vi "MT Demodulate CPM.vi"(0 "input complex waveform":T1={"t0"=0.0, "dt"=1.0, "Y"=[]} {"Y" format="%.3f"; "dt" format="%^.2e"; "t0" format="%.4f"}, 5 "CPM system parameters":T3={"samples per symbol (16)"=1, "symbol map"=[]}, 7 "matched filter coefficients":dbl[](array[numeric]) format="%.2f", 9 "synchronization parameters":T4 {"sync sequence" format="%.2f"}, 11 "error in (no error)":errorcluster, 12 "pulse shaping filter coefficients":dbl[](array[numeric]) format="%.2f", 13 "reset? (T)":bool=TRUE) -> (3 "detected complex waveform":T1 {"Y" format="%.3f"; "dt" format="%^.2e"; "t0" format="%.4f"}, 4 "recovered complex waveform":T1 {"Y" format="%.3f"; "dt" format="%^.2e"; "t0" format="%.4f"}, 6 "output bit stream":i8[](array[numeric]), 8 "measurements":T2 {"frequency drift (Hz)" format="%.2f"; "frequency offset (Hz)" format="%.2f"}, 10 "sync found index (symbols)":dbl format="%.4f", 15 "error out":errorcluster)   [LabVIEW 2020, in "niDMT.lvlib"]
doc: "Demodulates a continuous-phase modulation (CPM)-modulated complex baseband waveform and returns the time-aligned demodulated waveform, the demodulated information bit stream, and measurement results obtained during demodulation. This VI attempts to remove carrier and phase offset by locking to the carrier signal."
uses:
  <vilib>/addons/Modulation/niDMT.lvlib
  <vilib>/addons/Modulation/Analog/controls/Complex Data Waveform.ctl
  <vilib>/addons/Modulation/Digital/Support/Controls/CPM System Parameters.ctl
  <vilib>/addons/Modulation/Analog/MT Resample (Complex Cluster).vi
  <vilib>/addons/Modulation/Analog/support/Validators/mod_Fractional Resample Validate.vi
  <vilib>/addons/Modulation/Analog/support/Validators/mod_Check Flush State.vi
  <vilib>/addons/Modulation/Analog/support/mod_FractionalResampler.vi
  <vilib>/addons/Modulation/Analog/support/mod_Integer Rate Interpolation.vi
  <vilib>/addons/Modulation/Analog/support/Validators/mod_Validate Complex Waveform.vi
  <vilib>/addons/Modulation/Analog/support/mod_PerformResampling.vi
  <vilib>/addons/Modulation/Analog/support/Validators/mod_WFErrorHandler.vi
  <vilib>/addons/Modulation/Digital/Support/Common/mod_Truncate FIR Filter (real).vi
  <vilib>/Utility/error.llb/Error Cluster From Error Code.vi
  <vilib>/addons/Modulation/Analog/support/mod_Resampling Factors.vi
  <vilib>/addons/Modulation/Analog/support/mod_ResamplingFilter.vi
  <vilib>/addons/Modulation/Analog/support/mod_Generate Integer Interpolation Filter.vi
  <vilib>/addons/Modulation/niAMT.lvlib
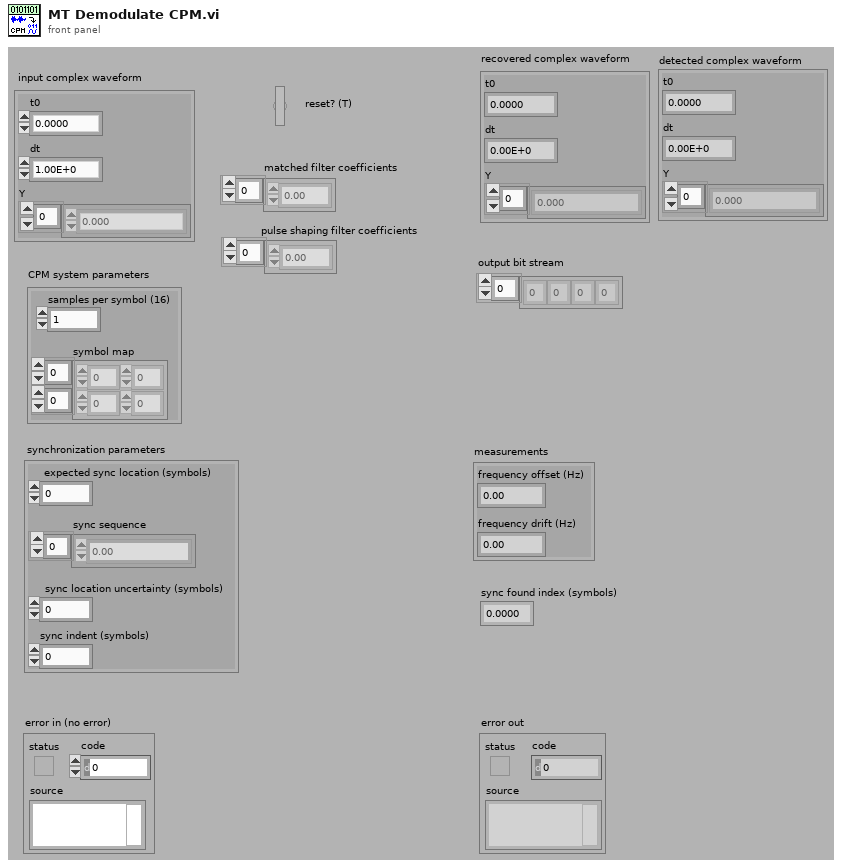
[diagram p1: front panel]
types:
  T1 = typedef "niAMT.lvlib/Complex Data Waveform.ctl" = cluster{"t0":dbl, "dt":dbl, "Y":cdb[]}
  T2 = cluster{"frequency offset (Hz)":dbl, "frequency drift (Hz)":dbl}
  T3 = typedef "niDMT.lvlib/CPM System Parameters.ctl" = cluster{"samples per symbol (16)":i32, "symbol map":dbl[][]}
  T4 = cluster{"expected sync location (symbols)":i32, "sync sequence":cdb[], "sync location uncertainty (symbols)":i32, "sync indent (symbols)":i32}
  T5 = enum16{"FSK", "PSK", "QAM", "MSK", "PAM", "ASK", "CPM"}
  T6 = cluster{"Frequency Estimate, Hz":dbl, "Frequency Drift, Hz":dbl}
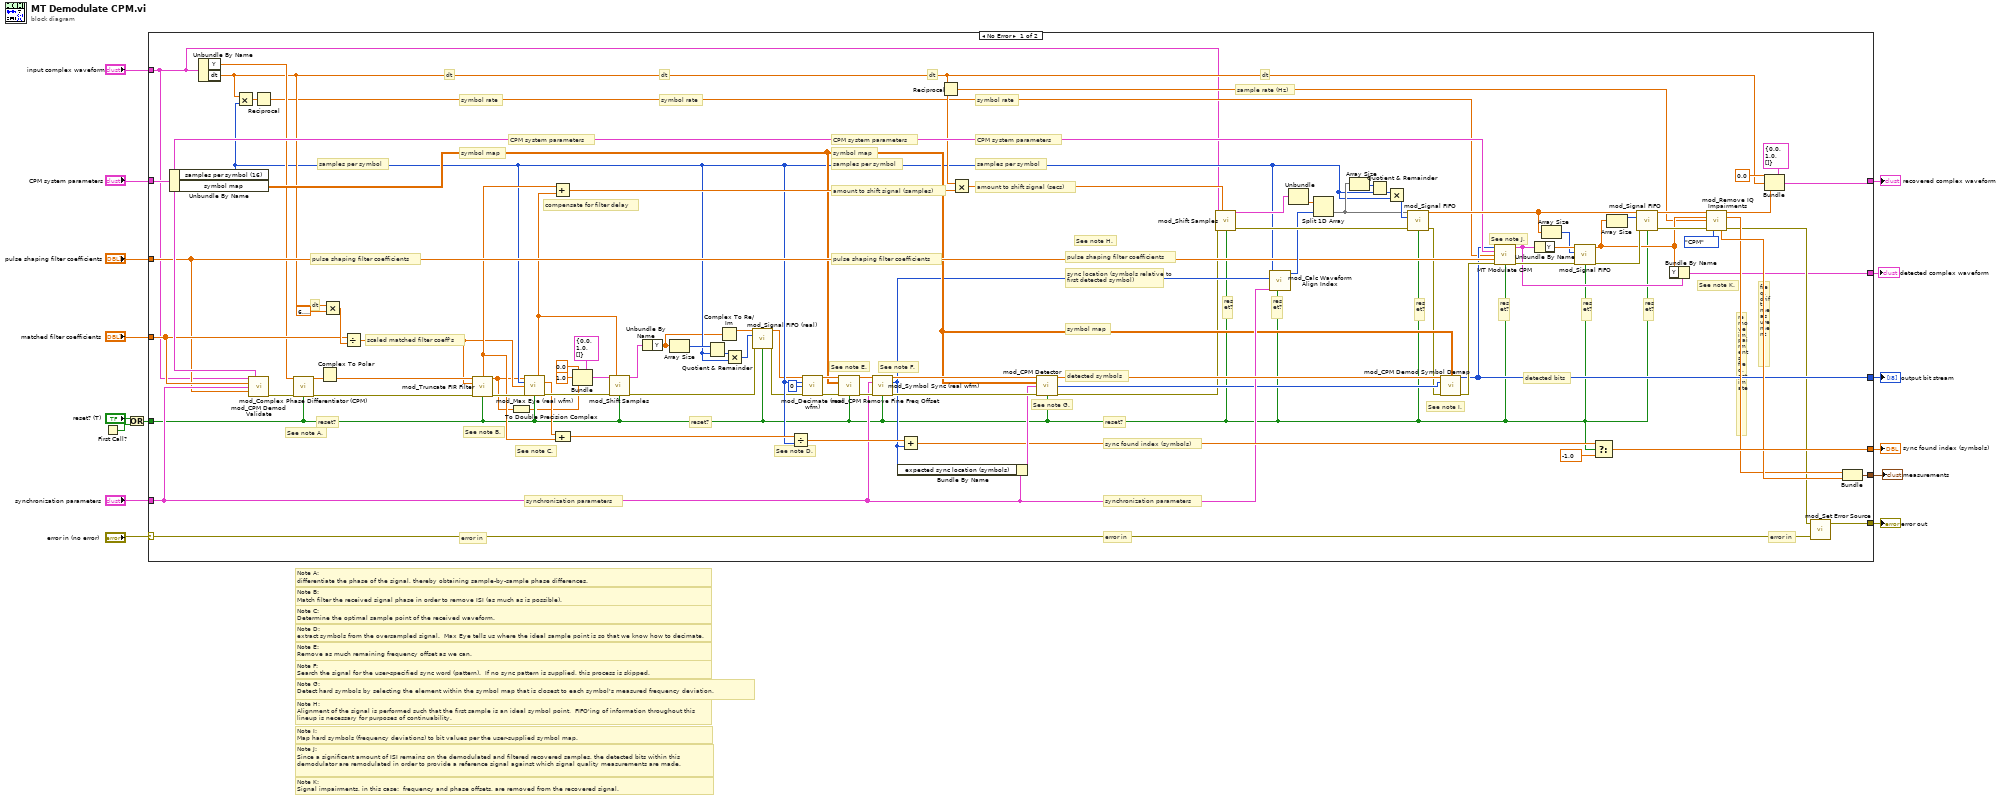
[diagram p0: block diagram]
diagram:
  # "Note K:\nSignal impairments, in this case:  frequency and phase offsets, are removed from the recovered signal."
  # "Note J:\nSince a significant amount of ISI remains on the demodulated and filtered recovered samples, the detected bits within this demodulator are remodulated in order to provide a reference signal against which signal quality measurements are made."
  # "Note I:\nMap hard symbols (frequency deviations) to bit values per the user-supplied symbol map."
  # "Note H:\nAlignment of the signal is performed such that the first sample is an ideal symbol point.  FIFO'ing of information throughout this \nlineup is necessary for purposes of continuability."
  # "Note G:\nDetect hard symbols by selecting the element within the symbol map that is closest to each symbol's measured frequency deviation."
  # "Note F:\nSearch the signal for the user-specified sync word (pattern).  If no sync pattern is supplied, this process is skipped."
  # "Note E:\nRemove as much remaining frequency offset as we can."
  # "Note D:\nextract symbols from the oversampled signal.  Max Eye tells us where the ideal sample point is so that we know how to decimate."
  # "Note C:\nDetermine the optimal sample point of the received waveform."
  # "Note B:\nMatch filter the received signal phase in order to remove ISI (as much as is possible)."
  # "Note A:\ndifferentiate the phase of the signal, thereby obtaining sample-by-sample phase differences."
  n1 = First Call?() -> (First Call?: T/F=w3:bool)
  n2 = Or(x="reset? (T)", y=w3) -> (x .or. y?=w5:bool)
  n3 = case shown="No Error" "error in (no error)" {
    selector: "error in (no error)" -> [w102 w108]
    tunnel: [w103 w108] -> w8
    tunnel: "synchronization parameters" -> [w59 _]
    tunnel: "matched filter coefficients" -> [w60 _]
    tunnel: "pulse shaping filter coefficients" -> [w58 _]
    tunnel: [w94 _] -> w9
    tunnel: "input complex waveform" -> [w17 _]
    tunnel: [w35 _] -> w10
    tunnel: [w105 _] -> w2
    tunnel: w5 -> [w29 _]
    tunnel: [w100 _] -> w6
    tunnel: "CPM system parameters" -> [w61 _]
    tunnel: [w25 _] -> w1
    frame No Error {
      # "See note K."
      # "See note J."
      # "See note I."
      # "See note H."
      # "See note G."
      # "See note F."
      # "See note E."
      # "See note D."
      # "See note C."
      # "See note B."
      # "See note A."
      # "reset?"
      # "freq. drift measurement"
      # "reset?"
      # "reset?"
      # "reset?"
      # "reset?"
      # "reset?"
      # "remove impairments freq. estimate"
      # "error in"
      # "detected bits"
      # "error in"
      # "synchronization parameters"
      # "error in"
      # "synchronization parameters"
      # "sync found index (symbols)"
      # "sample rate (Hz)"
      # "dt"
      # "reset?"
      # "reset?"
      # "reset?"
      # "detected symbols"
      # "sync location (symbols relative to first detected symbol)"
      # "pulse shaping filter coefficients"
      # "amount to shift signal (secs)"
      # "symbol map"
      # "symbol rate"
      # "dt"
      # "CPM system parameters"
      # "symbol map"
      # "samples per symbol"
      # "symbol rate"
      # "dt"
      # "CPM system parameters"
      # "samples per symbol"
      # "pulse shaping filter coefficients"
      # "amount to shift signal (samples)"
      # "scaled matched filter coeff's"
      # "pulse shaping filter coefficients"
      # "samples per symbol"
      # "compensate for filter delay"
      # "symbol map"
      # "CPM system parameters"
      # "dt"
      # "dt"
      # "symbol rate"
      n4 = Unbundle By Name(w61) -> ("samples per symbol (16)"=w38:i32, "symbol map"=w57:dbl[][])
      n5 = Unbundle By Name(w17) -> ("Y"=w45:cdb[], "dt"=w44:dbl)
      n6 = Multiply(x=w44, y=w38) -> (x*y=w106:dbl)
      n7 = call <vilib>:"mod_CPM Demod Validate.vi"("Input Complex Waveform"=w17, "CPM system parameters"=w61, "Matched Filter Coefficients"=w60, "Synchronization Parameters"=w59, "Pulse Shaping Filter Coefficients"=w58) -> ("error out"=w55:errorcluster)  [unwired: 10 out]
      n8 = Reciprocal(x=w106) -> (1/x=w34:dbl)
      n9 = call <vilib>:"mod_Complex Phase Differentiator (CPM).vi"("Signal In"=w45, "error in (no error)"=w55, "Reset? (T)"=w29) -> ("Signal Out"=w79:cdb[], "error out"=w68:errorcluster)  [unwired: 11 in]
      n10 = Complex To Polar(r * e^(i*theta)=w79) -> (theta=w67:dbl[])  [unwired: 1 out]
      n11 = Multiply(x=w44, y=6.283185307179586) -> (x*y=w70:dbl)
      n12 = Divide(x=w60, y=w70) -> (x/y=w42:dbl[])
      n13 = call-poly <vilib>:"mod_Truncate FIR Filter.vi"("Signal In"=w67, "Filter Coefficients"=w42, "error in (no error)"=w68, "Reset? (T)"=w29) -> ("Fractional Delay (samples)"=w43:dbl, "Signal Out"=w24:dbl[], "error out"=w77:errorcluster)  [unwired: 8 in, 1 out]
      n14 = To Double Precision Complex(1:w24) -> (0:w21:cdb[])
      n15 = call <vilib>:"mod_Max Eye (real wfm).vi"("Signal In"=w24, "Samples Per Symbol (16)"=w38, "Filter Coefficients"=w42, "error in (no error)"=w77, "Reset? (T)"=w29) -> ("Waveform Alignment Offset"=w46:dbl, "Optimal Offset (samples)"=w41:dbl, "error out"=w47:errorcluster)  [unwired: 6 in, 2 out]
      n16 = Add(x=w43, y=w46) -> (x+y=w69:dbl)
      n17 = Compound Arithmetic op=ADD(w41, w43) -> (w76:dbl)
      n18 = Bundle(cluster=T1 {"t0"=0.0, "dt"=1.0, "Y"=[]} ("data waveform"), "t0"=0.0, "dt"=1.0, "Y"=w21) -> (w51:T1)
      n19 = call <vilib>:"mod_Shift Samples.vi"("Input Complex Waveform"=w51, "Initial Sample Offset, sec"=w46, "error in (no error)"=w47, "Reset? (T)"=w29) -> ("Output Complex Waveform"=w40:T1, "error out"=w28:errorcluster)  [unwired: 10 in]
      n20 = Unbundle By Name(w40) -> ("Y"=w23:cdb[])
      n21 = Array Size(array=w23) -> (size(s)=w50:i32)
      n22 = Quotient & Remainder(x=w50, y=w38) -> (floor(x/y)=w49:i32)  [unwired: 1 out]
      n23 = Complex To Re/Im(x + iy=w23) -> (x=w22:dbl[])  [unwired: 1 out]
      n24 = Multiply(x=w49, y=w38) -> (x*y=w31:i32)
      n25 = call <vilib>:"mod_Signal FIFO (real).vi"("Signal In"=w22, "Output Length"=w31, "error in (no error)"=w28, "Reset? (T)"=w29) -> ("Signal Out"=w30:dbl[], "error out"=w27:errorcluster)  [unwired: 10 in]
      n26 = Divide(x=w76, y=w38) -> (x/y=w96:dbl)
      n27 = call <vilib>:"mod_Decimate (real wfm).vi"("Signal In"=w30, "Samples Per Symbol (16)"=w38, "Offset"=0, "error in (no error)"=w27) -> ("Signal Out"=w64:dbl[], "error out"=w66:errorcluster)  [unwired: 10 in]
      n28 = call <vilib>:"mod_CPM Remove Fine Freq Offset.vi"("Symbols"=w64, "Symbol Map"=w57, "error in (no error)"=w66, "Reset? (T)"=w29) -> ("Symbols"=w63:dbl[], "error out"=w65:errorcluster)  [unwired: 10 out]
      n29 = call <vilib>:"mod_Symbol Sync (real wfm).vi"("Signal In"=w63, "Synchronization Parameters"=w59, "error in (no error)"=w65, "Reset? (T)"=w29) -> ("Signal Out"=w78:dbl[], "Sync Location (symbols)"=w39:i32, "error out"=w107:errorcluster)  [unwired: 9 in]
      n30 = Bundle By Name(cluster=w59, "expected sync location (symbols)"=w39) -> (w104:T4)
      n31 = Add(x=w96, y=w39) -> (x+y=w93:dbl)
      n32 = Reciprocal(x=w44) -> (1/x=w18:dbl)
      n33 = Multiply(x=w44, y=w69) -> (x*y=w82:dbl)
      n34 = call <vilib>:"mod_CPM Detector.vi"("Symbols"=w78, "Symbol Map"=w57, "Synchronization Parameters"=w104, "error in (no error)"=w107, "reset ? (T/F)"=w29) -> ("Detected Symbols"=w71:dbl[], "detected modulation indices"=w54:i32[], "error out"=w16:errorcluster)  [unwired: 8 out]
      n35 = call <vilib>:"mod_Shift Samples.vi"("Input Complex Waveform"=w17, "Initial Sample Offset, sec"=w82, "error in (no error)"=w16, "Reset? (T)"=w29) -> ("Output Complex Waveform"=w75:T1, "error out"=w88:errorcluster)  [unwired: 10 in]
      n36 = call <vilib>:"mod_Calc Waveform Align Index.vi"("Reset? (T)"=w29, "Synchronization Parameters"=w59, "Sync Location, symbols"=w39, "Samples Per Symbol (16)"=w38) -> ("align index, samples"=w81:i32)  [unwired: 7 out]
      n37 = Unbundle(w75) -> ("Y"=w80:cdb[])  [unwired: 2 out]
      n38 = Split 1D Array(array=w80, index=w81) -> (second subarray=w89:cdb[])  [unwired: 1 out]
      n39 = Array Size(array=w89) -> (size(s)=w92:i32)
      n40 = Quotient & Remainder(x=w92, y=w38) -> (floor(x/y)=w91:i32)  [unwired: 1 out]
      n41 = Multiply(x=w91, y=w38) -> (x*y=w90:i32)
      n42 = call <vilib>:"mod_Signal FIFO.vi"("Signal In"=w89, "Output Length"=w90, "error in (no error)"=w88, "Reset? (T)"=w29) -> ("Signal Out"=w73:cdb[], "error out"=w37:errorcluster)  [unwired: 10 out]
      n43 = call <vilib>:"mod_CPM Demod Symbol Demap.vi"("Symbols In"=w71, "Symbol Map"=w57, "input modulation indices"=w54, "error in (no error)"=w37) -> ("Bits Out"=w35:i8[], "error out"=w36:errorcluster)  [unwired: 1 in, 9 out]
      n44 = call <vilib>:"MT Modulate CPM.vi"("input bit stream"=w35, "CPM system parameters"=w61, "symbol rate (Hz)"=w34, "pulse shaping filter coefficients"=w58, "error in (no error)"=w36, "reset? (T)"=w29) -> ("output complex waveform"=w33:T1, "error out"=w98:errorcluster)  [unwired: 1 in, 7 out]
      n45 = Unbundle By Name(w33) -> ("Y"=w99:cdb[])
      n46 = Array Size(array=w73) -> (size(s)=w97:i32)
      n47 = call <vilib>:"mod_Signal FIFO.vi"("Signal In"=w99, "Output Length"=w97, "error in (no error)"=w98, "Reset? (T)"=w29) -> ("Signal Out"=w32:cdb[], "error out"=w85:errorcluster)  [unwired: 10 out]
      n48 = Select(t=w93, s=w29, f=-1.0) -> (s? t:f=w94:dbl)
      n49 = Array Size(array=w32) -> (size(s)=w86:i32)
      n50 = call <vilib>:"mod_Signal FIFO.vi"("Signal In"=w73, "Output Length"=w86, "error in (no error)"=w85, "Reset? (T)"=w29) -> ("Signal Out"=w83:cdb[], "error out"=w84:errorcluster)  [unwired: 10 out]
      n51 = Bundle By Name(cluster=w33, "Y"=w32) -> (w25:T1)
      n52 = call <vilib>:"mod_Remove IQ Impairments.vi"("Received Signal In"=w83, "Reference Signal"=w32, "Signal Rate, Hz"=w18, "error in (no error)"=w84, "Modulation Type"=T5."CPM") -> ("Received Signal Out"=w101:cdb[], "Frequency Estimate, Hz"=w72:dbl, "Frequency Drift, Hz"=w87:dbl, "error out"=w26:errorcluster)  [unwired: 7 out]
      n53 = Bundle(cluster=T1 {"t0"=0.0, "dt"=1.0, "Y"=[]} ("data waveform"), "t0"=0.0, "dt"=w44, "Y"=w101) -> (w100:T1)
      n54 = call <vilib>:"mod_Set Error Source.vi"("initial error in (no error)"=w102, "final error in (no error)"=w26) -> ("error out"=w103:errorcluster)  [unwired: 3 out]
      n55 = Bundle("Frequency Estimate, Hz"=w72, "Frequency Drift, Hz"=w87) -> (w105:T6)  [unwired: 1 out]
    }
    frame Error {
    }
  }
  "error out" <- w8
  "sync found index (symbols)" <- w9
  "output bit stream" <- w10
  "recovered complex waveform" <- w6
  "measurements" <- w2
  "detected complex waveform" <- w1
